vi "Build Shared Variable Arrays.vi"(8 "error in (no error)":errorcluster, 10 "IP Address":string, 11 "Channel Ref in":T2 format="%.0x") -> (0 "error out":errorcluster, 1 "Channel Type":T1, 2 "Shared Variable URL":string, 3 "Channel Ref out":T2 format="%.0x")   [LabVIEW 2015, in "Shared Variable Custom Device.lvlib"]
uses:
  Shared Variable Custom Device.lvlib
  <vilib>/NI Veristand/Custom Device API/Custom Device Item Ref.ctl
  <vilib>/Utility/VariantDataType/Type.ctl
  <vilib>/NI Veristand/Custom Device API/Custom Device API.lvlib
  <vilib>/Utility/VariantDataType/VariantType.lvlib
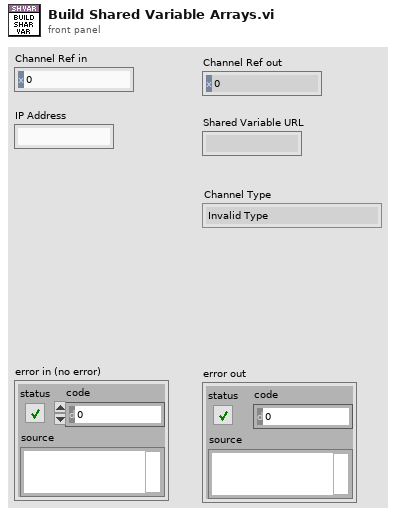
[diagram p1: front panel]
types:
  T1 = typedef "VariantType.lvlib/Type.ctl" = enum8{"Invalid Type", "Void", "I8", "I16", "I32", "I64", "U8", "U16", "U32", "U64", "Single Float", "Double Float", "Extended Float", "Single Complex", "Double Complex", "Extended Complex", "Enum U8", "Enum U16", "Enum U32", "Enum U64", "Single Float With Unit", "Double Float With Unit", "Extended Float With Unit", "Single Complex with Unit", "Double Complex with Unit", "Extended Complex with Unit", "Boolean", "String", "Path", "Picture", "Tag", "Array", "Cluster", "Variant", "LV Variant", "Waveform", "Timestamp", "Digital Waveform", "Digital Data", "ExpressData", "Refnum", "External Data", "VI", "Poly VI", "LabVIEW Class Instance", "Fixed Point"}
  T2 = typedef "Custom Device API.lvlib/Custom Device Item Ref.ctl" = u64
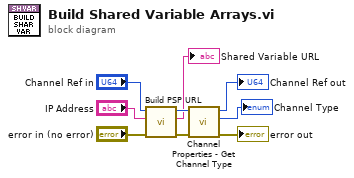
[diagram p0: block diagram]
diagram:
  n1 = call "Build PSP URL.vi"("error in (no error)"="error in (no error)", "IP Address"="IP Address", "Channel Ref in"="Channel Ref in") -> ("error out"=w7:errorcluster, "Shared Variable URL"=→"Shared Variable URL":string, "Channel Ref out"=w6:T2)  [unwired: 6 in]
  n2 = call "Channel Properties - Get Channel Type.vi"("error in (no error)"=w7, "Channel Ref in"=w6) -> ("error out"=→"error out":errorcluster, "Channel Type"=→"Channel Type":T1, "Channel Ref out"=→"Channel Ref out":T2)  [unwired: 7 in]
